vi "PDT Batch.vi"() -> ()   [LabVIEW 2018]
uses:
  <vilib>/Utility/file.llb/Read Delimited Spreadsheet (string).vi
panel:
  out "Headers":string[](array[string])
  in  "Batch PDT FilePath":path
  in  "PDT *.csv FilePath":path=path "C:/Users/dev/Downloads/PDT.csv"
  out "String":string
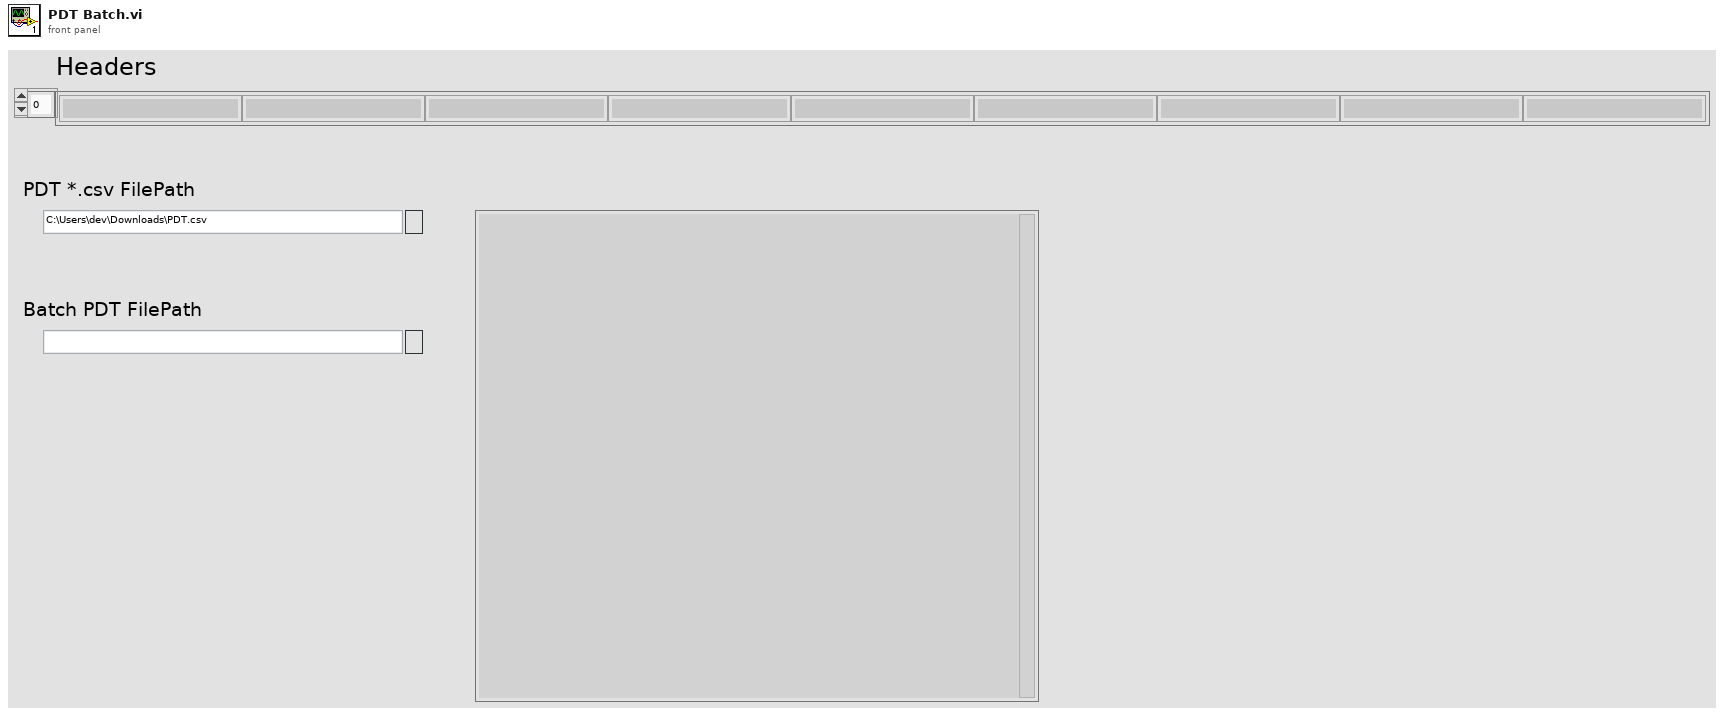
[diagram p1: front panel]
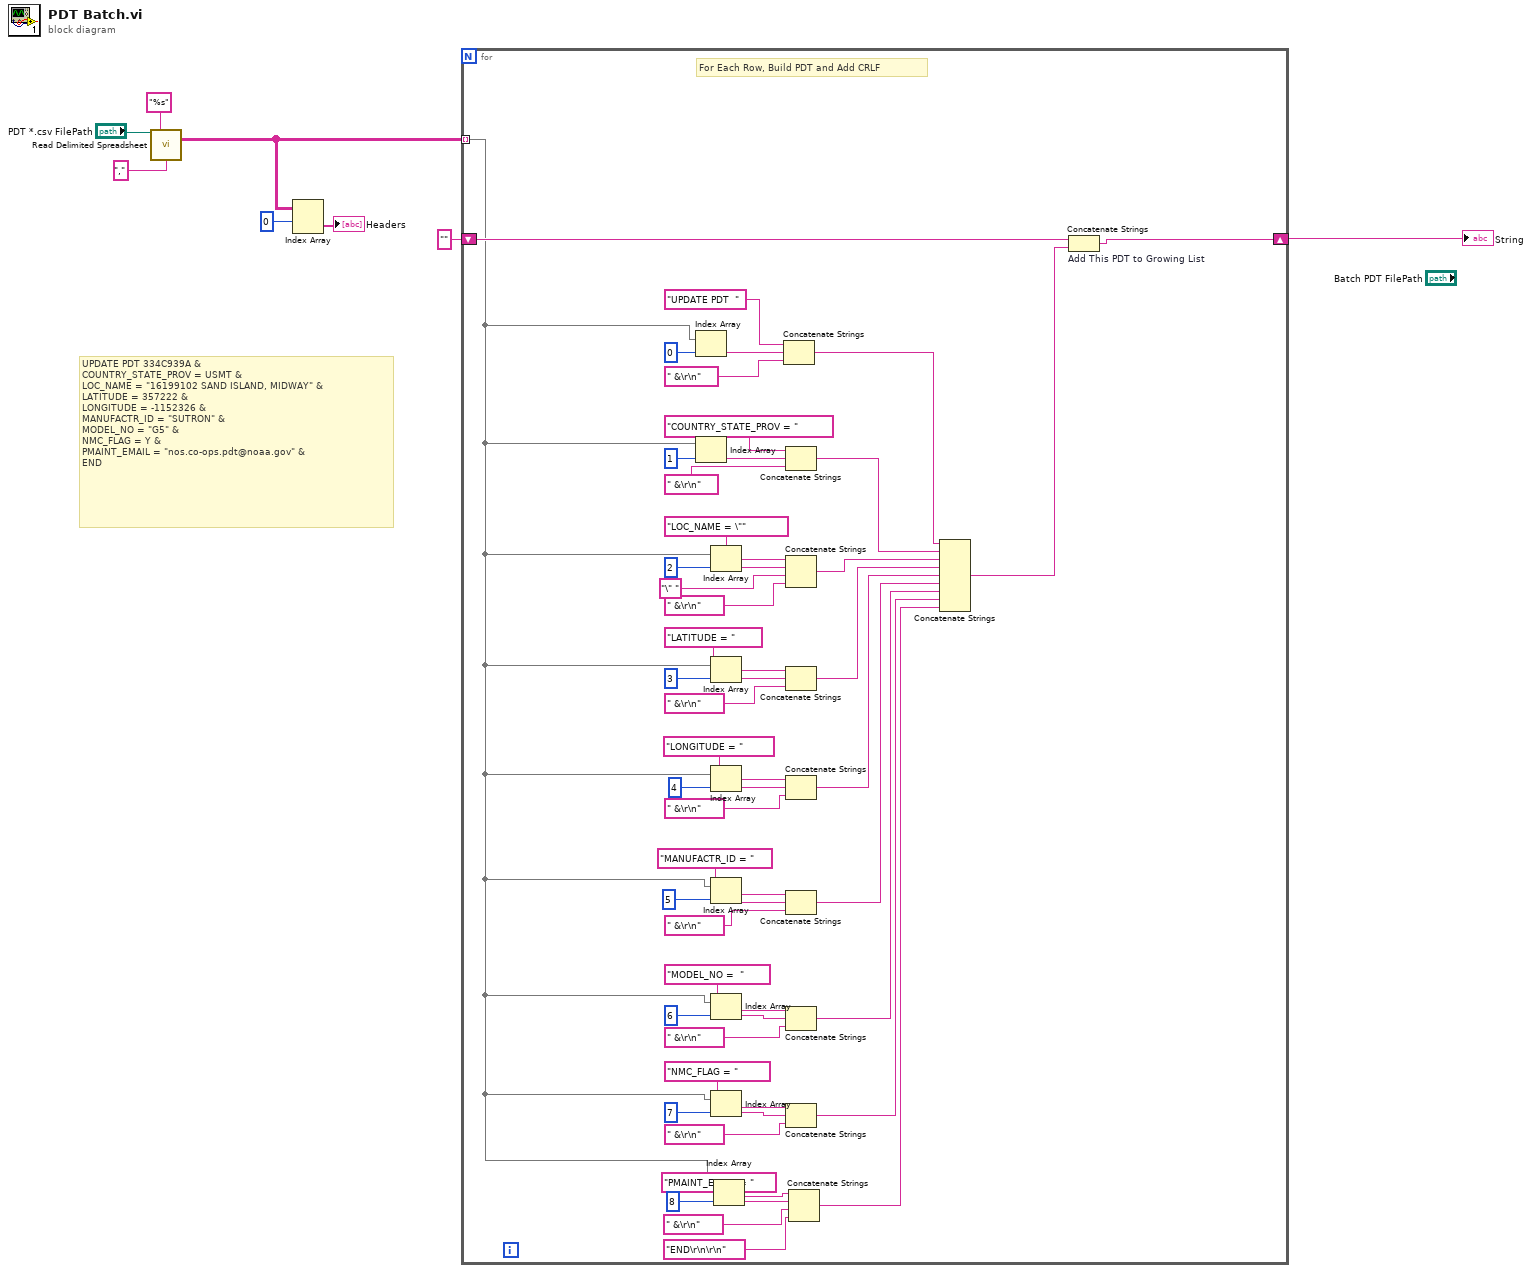
[diagram p0: block diagram]
diagram:
  # "UPDATE PDT 334C939A &\nCOUNTRY_STATE_PROV = USMT & \nLOC_NAME = \"16199102 SAND ISLAND, MIDWAY\" & \nLATITUDE = 357222 &\nLONGITUDE = -1152326 &\nMANUFACTR_ID = \"SUTRON\" & \nMODEL_NO = \"G5\" &\nNMC_FLAG = Y &\nPMAINT_EMAIL = \"nos.co-ops.pdt@noaa.gov\" & \nEND"
  n1 = call-poly <vilib>:"Read Delimited Spreadsheet.vi"("file path (dialog if empty)"="PDT *.csv FilePath", "format (%s)"="%s" ("format (%.3f)"), "delimiter (\\t)"="," ("delimiter (\\t)")) -> ("all rows"=w2:string[][])  [unwired: 7 in, 5 out]
  n2 = Index Array(array=w2, index (row)=0 ("index")) -> (element=→"Headers":string[])  [unwired: 1 in]
  n3 = for {
    tunnel: w2 -> [w11] mode=indexing
    shift-right: [w44] -> w5
    shift-left: "" -> [w43]
    # "For Each Row, Build PDT and Add CRLF"
    n4 = Index Array(array=w11, index=0) -> (element=w57:string)
    n5 = Index Array(array=w11, index=1) -> (element=w36:string)
    n6 = Index Array(array=w11, index=2) -> (element=w55:string)
    n7 = Index Array(array=w11, index=3) -> (element=w32:string)
    n8 = Index Array(array=w11, index=4) -> (element=w29:string)
    n9 = Index Array(array=w11, index=5) -> (element=w40:string)
    n10 = Index Array(array=w11, index=6) -> (element=w52:string)
    n11 = Index Array(array=w11, index=7) -> (element=w13:string)
    n12 = Index Array(array=w11, index=8) -> (element=w49:string)
    n13 = Concatenate Strings("UPDATE PDT  ", w57, " &\r\n") -> (w38:string)
    n14 = Concatenate Strings("COUNTRY_STATE_PROV = ", w36, " &\r\n") -> (w34:string)
    n15 = Concatenate Strings("LOC_NAME = \"", w55, "\" ", " &\r\n") -> (w46:string)
    n16 = Concatenate Strings("LATITUDE = ", w32, " &\r\n") -> (w27:string)
    n17 = Concatenate Strings("LONGITUDE = ", w29, " &\r\n") -> (w26:string)
    n18 = Concatenate Strings("MANUFACTR_ID = ", w40, " &\r\n") -> (w25:string)
    n19 = Concatenate Strings("MODEL_NO =  ", w52, " &\r\n") -> (w17:string)
    n20 = Concatenate Strings("NMC_FLAG = ", w13, " &\r\n") -> (w9:string)
    n21 = Concatenate Strings("PMAINT_EMAIL = ", w49, " &\r\n", "END\r\n\r\n") -> (w10:string)
    n22 = Concatenate Strings(w38, w34, w46, w27, w26, w25, w17, w9, w10) -> (w45:string)
    n23 = Concatenate Strings "Add This PDT to Growing List"(w43, w45) -> (w44:string)
  }
  "String" <- w5
